vi "Error_To_Warning.vi"(6 "Error Codes to be handled as warnings":i32[](array[numeric]), 8 "error in":errorcluster) -> (0 "error out":errorcluster)   [LabVIEW 2017]
doc: "This VI turns errors into warnings. It searches for an error code in the input array and if the input error code is found in the input errors array, it turns the input error into a warning."
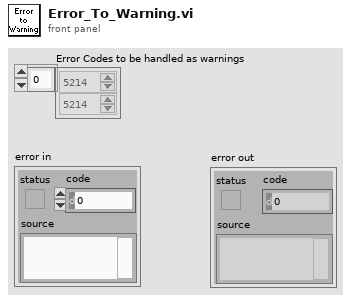
[diagram p1: front panel]
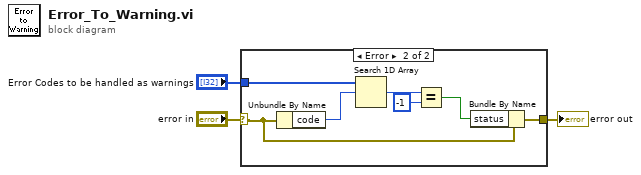
[diagram p0: block diagram]
diagram:
  n1 = case shown="Error" "error in" {
    selector: "error in" -> [w4 w11]
    tunnel: [w4 w10] -> w2
    tunnel: "Error Codes to be handled as warnings" -> [_ w9]
    frame No Error {
    }
    frame Error {
      n2 = Unbundle By Name(w11) -> ("code"=w8:i32)
      n3 = Search 1D Array(1D array=w9, element=w8) -> (index of element=w7:i32)  [unwired: 1 in]
      n4 = Equal?(x=w7, y=-1) -> (x = y?=w5:bool)
      n5 = Bundle By Name(cluster=w11, "status"=w5) -> (w10:errorcluster)
    }
  }
  "error out" <- w2
